vi "Vehicle Position Simulation View.vi"(8 "error in (no error)":errorcluster, 11 "View Model":T2) -> (0 "error out":errorcluster, 3 "View Model":T2)   [LabVIEW 2017]
doc: "The interface via which the user is able to simulate the travel of a vehicle in the car wash enclosure during a wash cycle.\n[Covers: UI4]"
uses:
  View Model/Controls/View Model.ctl
  View Model/Controls/Shared Model.ctl
  Error Handler/Controls/Error Model.ctl
  Error Handler/Controls/Error Data.ctl
  Error Handler/Controls/Error Level.ctl
  Configuration/Controls/Config Model.ctl
  Configuration/Controls/Config Record.ctl
  Configuration/Controls/Config Data.ctl
  Configuration/Controls/Config Command.ctl
  Controller/Controls/Controler Model.ctl
  Entry Console View/Controls/Entry Console - Wash Steps.ctl
  Controller/Controls/Controller - Event.ctl
  Controller/Controls/Controller - Commands.ctl
  Controller/Controls/Controller - Overhead.ctl
  Controller/Controls/Controller - States.ctl
  Controller/Controls/Controller - Wash Step.ctl
  Controls/Vehicle - Station Enum.ctl
  Controls/Vehicle - Station Slider.ctl
panel:
  in  "Vehicle PosSim":T1 caption="Vehicle Position Simulation" max=4 step=1 scale=0.0..4.0
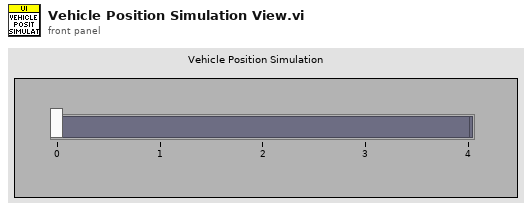
[diagram p1: front panel]
types:
  T1 = typedef "Vehicle - Station Slider.ctl" = u8
  T2 = typedef "View Model.ctl" = cluster{"Shared Model":T3, "Error Model":T4, "Config Model":T5, "Controler Model":T6}
  T3 = typedef "Shared Model.ctl" = cluster{"Stop":refnum<user-event>, "Stop DVR":refnum<data-value>}
  T4 = typedef "Error Model.ctl" = cluster{"Error":refnum<user-event>}
  T5 = typedef "Config Model.ctl" = cluster{"Config Recs DVR":refnum<data-value>, "Config Data":refnum<user-event>, "Config Lock":refnum<user-event>, "Config Lock DVR":refnum<data-value>}
  T6 = typedef "Controler Model.ctl" = cluster{"Wash Step Exec":refnum<user-event>, "Wash Step Complete":refnum<user-event>, "Wash Cycle Complete":refnum<user-event>, "Wash Cycle Start":refnum<user-event>, "Vehicle Out of Position":refnum<user-event>, "Command":refnum<user-event>, "Overhead DVR":refnum<data-value>, "Start Wash Step":refnum<user-event>, "Station Change":refnum<user-event>}
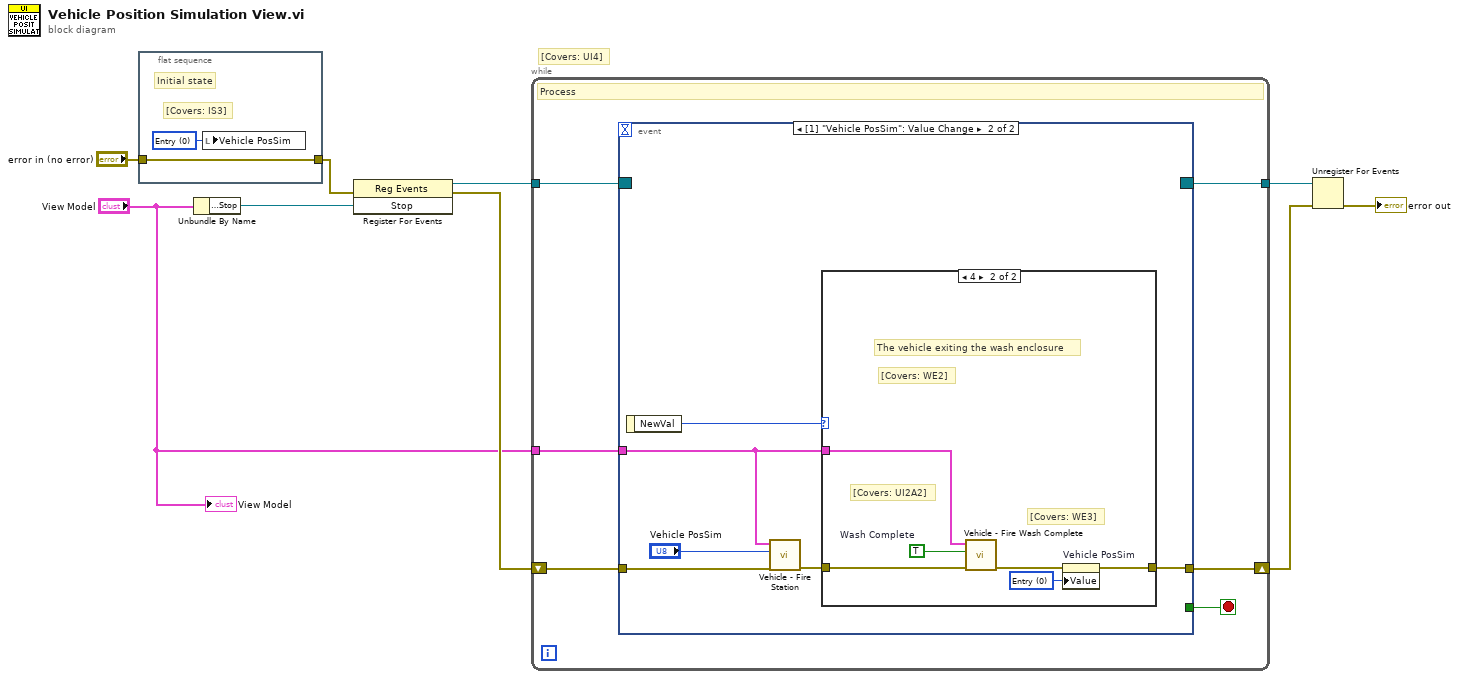
[diagram p0: block diagram]
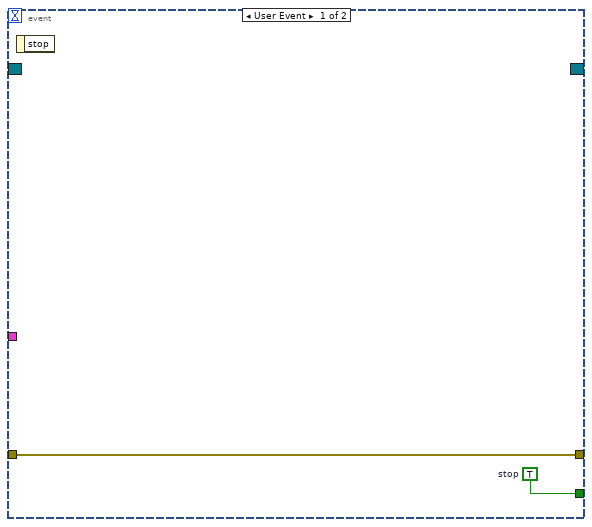
[diagram p2: hidden frame]
diagram:
  # "[Covers: UI4]"
  n1 = flat-sequence {
    tunnel: "error in (no error)" -> [w10]
    tunnel: [w10] -> w1
    frame #0 {
      w11 = T1 0 items=["Entry", "Station1", "Station2", "Station3", "Exit"] ("Vehicle PosSim")
      # "[Covers: IS3]"
      # "Initial state"
      n2 = local write "Vehicle PosSim"(w11) -> ()
    }
  }
  n3 = Unbundle By Name("View Model") -> ("Shared Model.Stop"=w9:refnum<user-event>)
  n4 = register-events(error in=w1, w9) -> (reference out=w8:refnum<event-registration>, error out=w7:errorcluster)  [unwired: 1 in]
  n5 = while {
    tunnel: w8 -> [w17]
    shift-right: [w15] -> w5
    shift-left: w7 -> [w16]
    tunnel: [w13] -> w6
    tunnel: "View Model" -> [w12]
    stop <- w14 stop-if-true
    # "Process"
    n6 = event shown="[1] \"Vehicle PosSim\": Value Change" {
      selector: w17 -> [_ _]
      dyn-events: [_ _] -> w13
      timeout: _ -> [_ _]
      tunnel: w16 -> [w19 w25]
      tunnel: [w19 w22] -> w15
      tunnel: [w18 _] -> w14
      tunnel: w12 -> [_ w21]
      event User Event {
        w18 = TRUE  # stop
        n7 = event-data() -> ()  [unwired: 1 in, 1 out]
      }
      event Value Change {
        n8 = event-data() -> ("NewVal"=w24:T1)  [unwired: 1 in]
        n9 = call "Vehicle - Fire Station.vi"("error in (no error)"=w25, "Vehicle PosSim"="Vehicle PosSim", "View Model"=w21) -> ("error out"=w23:errorcluster)  [unwired: 7 in, 1 out]
        n10 = case shown="4" w24 {
          tunnel: w23 -> [w26 w32]
          tunnel: [w26 w28] -> w22
          tunnel: w21 -> [_ w31]
          frame Default {
          }
          frame 4 {
            w27 = T1 0 items=["Entry", "Station1", "Station2", "Station3", "Exit"] ("Vehicle PosSim")
            w30 = TRUE  # Wash Complete
            # "[Covers: WE2]"
            # "[Covers: WE3]"
            # "[Covers: UI2A2]"
            # "The vehicle exiting the wash enclosure"
            n11 = call "Vehicle - Fire Wash Complete.vi"("error in (no error)"=w32, "Wash Complete"=w30, "View Model"=w31) -> ("error out"=w29:errorcluster)  [unwired: 7 in, 1 out]
            n12 = property on="Vehicle PosSim" class="Slide (strict)"(error in=w29, "Value"=w27) -> (error out=w28:errorcluster)  [unwired: 1 in, 1 out]
          }
        }
      }
    }
  }
  n13 = Unregister For Events(event registration refnum=w6, error in=w5) -> (error out=→"error out":errorcluster)
  "View Model" <- "View Model"
